vi "AddGlyphtoGManager.vi"(8 "error in":errorcluster, 10 "glyph manager":T1, 11 "CEF_Node in":refnum<class "CEF_Node.lvclass">) -> (0 "error out":errorcluster, 2 "glyph manager out":T1, 3 "CEF_Node out":refnum<class "CEF_Node.lvclass">)   [LabVIEW 2025, in "CEF.lvlib" / "CEF_Node.lvclass"]
doc: "Copyright 2017 National Instruments Corporation\n\nLicensed under the Apache License, Version 2.0 (the \"License\"); you may not use this file except in compliance with the License. You may obtain a copy of the License at http://www.apache.org/licenses/LICENSE-2.0\nUnless required by applicable law or agreed to in writing, software distributed under the License is distributed on an \"AS IS\" BASIS, WITHOUT WARRANTIES OR CONDITIONS OF ANY KIND, either express or implied. See the License for the specific language governing permissions and limitations under the License."
uses:
  CEF_Node.lvclass
  glyph manager/glyph manager.ctl
  <vilib>/picture/picture.llb/imagedata.ctl
  CEF.lvlib
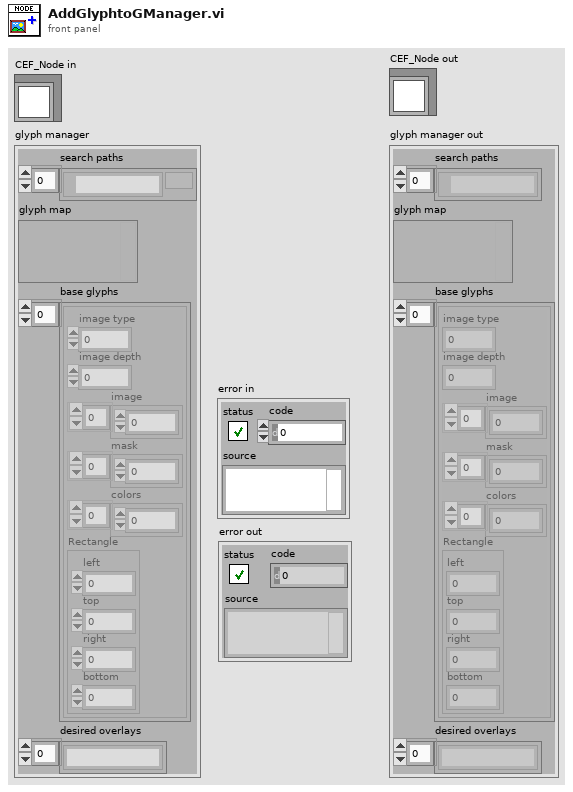
[diagram p1: front panel]
types:
  T1 = typedef "CEF.lvlib/glyph manager.ctl" = cluster{"search paths":path[], "glyph map":variant, "base glyphs":T2[], "desired overlays":string[]}
  T2 = typedef "imagedata.ctl" = cluster{"image type":i32, "image depth":i32, "image":u8[], "mask":u8[], "colors":u32[], "Rectangle":cluster{"left":i16, "top":i16, "right":i16, "bottom":i16}}
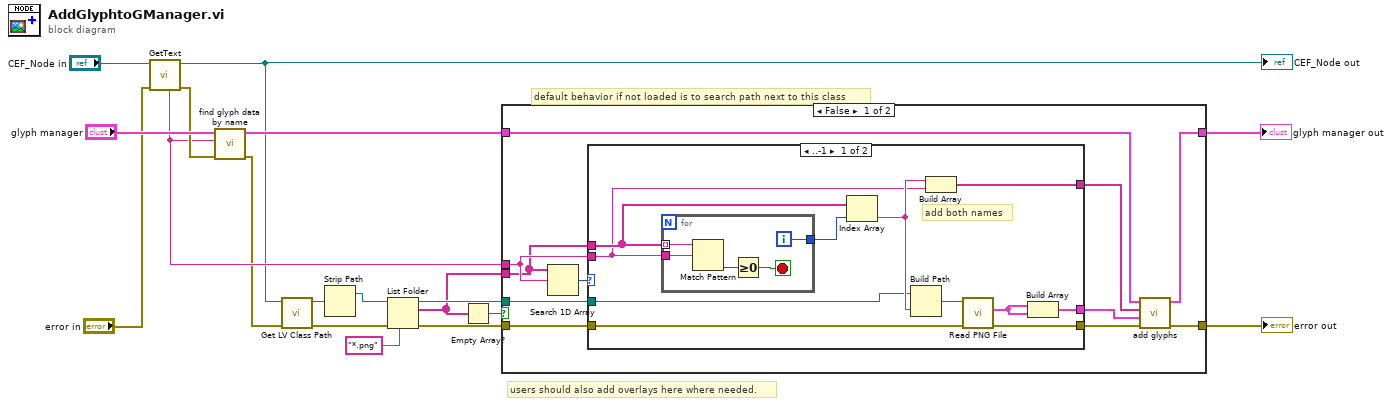
[diagram p0: block diagram]
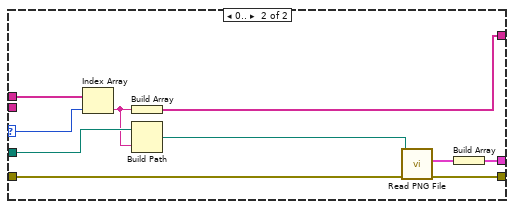
[diagram p2: hidden frame]
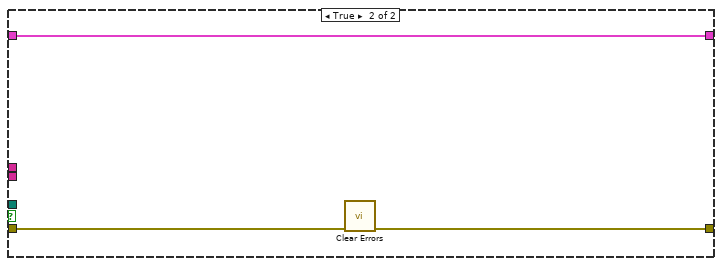
[diagram p3: hidden frame]
diagram:
  # "default behavior if not loaded is to search path next to this class"
  # "users should also add overlays here where needed."
  n1 = call-dynamic "GetText.vi"("error in"="error in", "CEF_Node in"="CEF_Node in") -> ("error out"=w12:errorcluster, "CEF_Node out"=w2:refnum<class "CEF_Node.lvclass">, "glyph"=w11:string)  [unwired: 5 in, 2 out]
  "CEF_Node out" <- w2
  n2 = call "find glyph data by name.vi"("error in"=w12, "name"=w11, "glyph manager in"="glyph manager") -> ("error out"=w1:errorcluster, "glyph manager out"=w15:T1)  [unwired: 5 in, 2 out]
  n3 = call <vilib>:"Get LV Class Path.vi"("error in (no error)"=w1, "object"=w2) -> ("error out"=w9:errorcluster, "class path"=w10:path)  [unwired: 8 in]
  n4 = Strip Path(path=w10) -> (stripped path=w8:path)  [unwired: 1 out]
  n5 = List Folder(path=w8, pattern="*.png", error in=w9) -> (path out=w6:path, filenames=w4:string[], error out=w5:errorcluster)  [unwired: 1 in, 1 out]
  n6 = Empty Array?(array=w4) -> (empty?=w3:bool)
  n7 = case shown="False" w3 {
    tunnel: w6 -> [w28 _]
    tunnel: w5 -> [w27 w57]
    tunnel: [w25 w56] -> w16
    tunnel: [w24 w58] -> w14
    tunnel: w15 -> [w23 w58]
    tunnel: w11 -> [w20 _]
    tunnel: w4 -> [w19 _]
    frame False {
      n8 = Search 1D Array(1D array=w19, element=w20) -> (index of element=w29:i32)  [unwired: 1 in]
      n9 = case shown="..-1" w29 {
        selector: w29 -> [_ w54]
        tunnel: w28 -> [w38 w53]
        tunnel: w19 -> [w37 w55]
        tunnel: w27 -> [w35 w51]
        tunnel: [w31 w48] -> w26
        tunnel: [w32 w47] -> w22
        tunnel: [w34 w46] -> w21
        tunnel: w20 -> [w30 _]
        frame ..-1 {
          # "add both names"
          n10 = for {
            tunnel: w37 -> [w45] mode=indexing
            tunnel: w30 -> [w44]
            tunnel: [w41] -> w36
            i -> [w41]
            stop <- w42 stop-if-true
            n11 = Match Pattern(string=w45, regular expression=w44) -> (offset past match=w43:i32)  [unwired: 1 in, 3 out]
            n12 = Greater Or Equal To 0?(x=w43) -> (x >= 0?=w42:bool)
          }
          n13 = Index Array(array=w37, index=w36) -> (element=w40:string)
          n14 = Build Path(base path=w38, name or relative path=w40) -> (appended path=w39:path)
          n15 = Build Array(w40, w30) -> (w32:string[])
          n16 = call <vilib>:"Read PNG File.vi"("error in (no error)"=w35, "path to PNG file"=w39) -> ("error out"=w31:errorcluster, "image data"=w33:T2)  [unwired: 7 in, 1 out]
          n17 = Build Array(w33, w33) -> (w34:T2[])
        }
        frame 0.. {
          n18 = Index Array(array=w55, index=w54) -> (element=w52:string)
          n19 = Build Array(w52) -> (w47:string[])
          n20 = Build Path(base path=w53, name or relative path=w52) -> (appended path=w50:path)
          n21 = call <vilib>:"Read PNG File.vi"("error in (no error)"=w51, "path to PNG file"=w50) -> ("error out"=w48:errorcluster, "image data"=w49:T2)  [unwired: 7 in, 1 out]
          n22 = Build Array(w49) -> (w46:T2[])
        }
      }
      n23 = call "add glyphs.vi"("error in"=w26, "glyphs"=w21, "names"=w22, "glyph manager in"=w23) -> ("error out"=w25:errorcluster, "glyph manager out"=w24:T1)  [unwired: 6 in]
    }
    frame True {
      n24 = call <vilib>:"Clear Errors.vi"("error in (no error)"=w57) -> ("error out"=w56:errorcluster)  [unwired: 5 in, 1 out]
    }
  }
  "error out" <- w16
  "glyph manager out" <- w14
